vi "cs-scanning_v2.vi"() -> ()   [LabVIEW 2017]
uses:
  controls/boolean_info.ctl
  z-axis-params.ctl
  <vilib>/rvi/Emulation/niFpgaGetClockAttributes.vi
  <vilib>/rvi/Emulation/niFpgaSctlEmulationGetInTimedLoop.vi
  <vilib>/rvi/Emulation/niFpgaEmulationReportErrorSimple.vi
  <vilib>/rvi/Emulation/niFpgaProcessEmulError.vi
  <vilib>/rvi/eio/common/nirviEmuTemplateMethod_errors.vi
  <vilib>/rvi/Emulation/niFpgaEmulationIsFPGAContextNoSignature.vi
  <vilib>/rvi/DataTransferAndStorage/Container/Common/niFpgaContainerGetUniqueNameForEmu.vi
  <vilib>/rvi/Memory/Memory_Emulation/niFpgaMemoryEmulationCacheClearOnFirstRun.vi
  <vilib>/rvi/Memory/Memory_Emulation/nirvimemoryEmulationManagerCache_MakeExclusive.vi
  <vilib>/rvi/Memory/Memory_Emulation/niFpgaMemoryEmulationValidateCache.vi
  <vilib>/rvi/Memory/Memory_Emulation/nirvimemoryEmulationManagerCache_InsertValue.vi
  <vilib>/Utility/error.llb/Clear Errors.vi
  <vilib>/rvi/Memory/Memory_Emulation/nirvimemoryEmulationManagerCache_ReleaseExclusive.vi
  <vilib>/rvi/Memory/Memory_Emulation/nirvimemoryEmulationManagerCache_GetValue.vi
  <vilib>/rvi/Memory/Memory_Emulation/nirvimemoryEmulationManagerCache_SetValue.vi
  <vilib>/rvi/Emulation/niFpgaCriticalErrorInLSC.vi
  <vilib>/eio/EIONode/EIONode.xnode
  <vilib>/rvi/DataTransferAndStorage/Container/XNode/niFpgaContainer.xnode
  <vilib>/rvi/DataTransferAndStorage/Register/Emulation/niFpgaRegisterEmulation.vi
  FPGA-data-logging.lvlib
  libimaging-cs.lvlib
panel:
  out "stop_loops":bool
  out "xy_k":fxp<+/-,16,5>[](array[numeric])
  out "xy_ref":fxp<+/-,16,5>[](array[numeric])
  out "u_x saturated":bool
  out "u_y saturated":bool
  in  "Kiz_down":sgl format="%#_13g"
  in  "max_Z_settle_samples":i16
  in  "step_down_frac":fxp<+,8,1>
  out "state1-count":u64
  out "state5-count":u64
  out "state4-count":u64
  out "state3-count":u64
  out "state2-count":u64
  in  "collect all":bool
  in  "collect move":bool=TRUE
  out "iter":i32
  out "entity-index":i16
  in  "TsTicks":u32=1600
  in  "z-axis-params":T1={"TOL"=0.3, "ramp_rate"=0.0, "z_u_max"=5.0, "setpoint"=0.0, "Ki"=0.001, "Z_error_threshold"=0.0, "Z_settled_samples_threshold "=0, "z_UP"=0.0, "zup_N"=0, "TF Order"=2, "Num"=[-0.00254, 0.000408, 0.00295, 0.0, 0.0, 0.0, 0.0, 0.0, 0.0], "Den"=[0.982758, -1.98194, 1.0, 0.0, 0.0, 0.0, 0.0, 0.0, 0.0]} {"Z_error_threshold" format="%#_13g"; "ramp_rate" format="%#_13g"; "TOL" format="%#_13g"}
  out "number-settled-samples-Z":i16
  out "Current Case":u8
  out "boolean \nindicators":T2
  out "z-u(k)":sgl
  in  "ABORT":bool
  out "read fifo timeout":bool
  in  "numEntities":i16
  in  "init Z up":fxp<+/-,16,5>
  in  "trigger-0":bool
  out "number-settled-samples-y":i16
  out "number-settled-samples-x":i16
  in  "xy-error-threshold":sgl format="%#_13g"
  in  "settled-samples\nthreshold":i16
  in  "Ki-xy":sgl=0.001 format="%#_13g"
  in  "xy-bound":sgl
  in  "initial case":u8
  # "- If collect all = fasle and collect move = false,\nwe only collect measurement data.\n- If collect all = false, and collect move = true,\nwe collect measurement and move data.\n- If collect all = true, we collect everything."
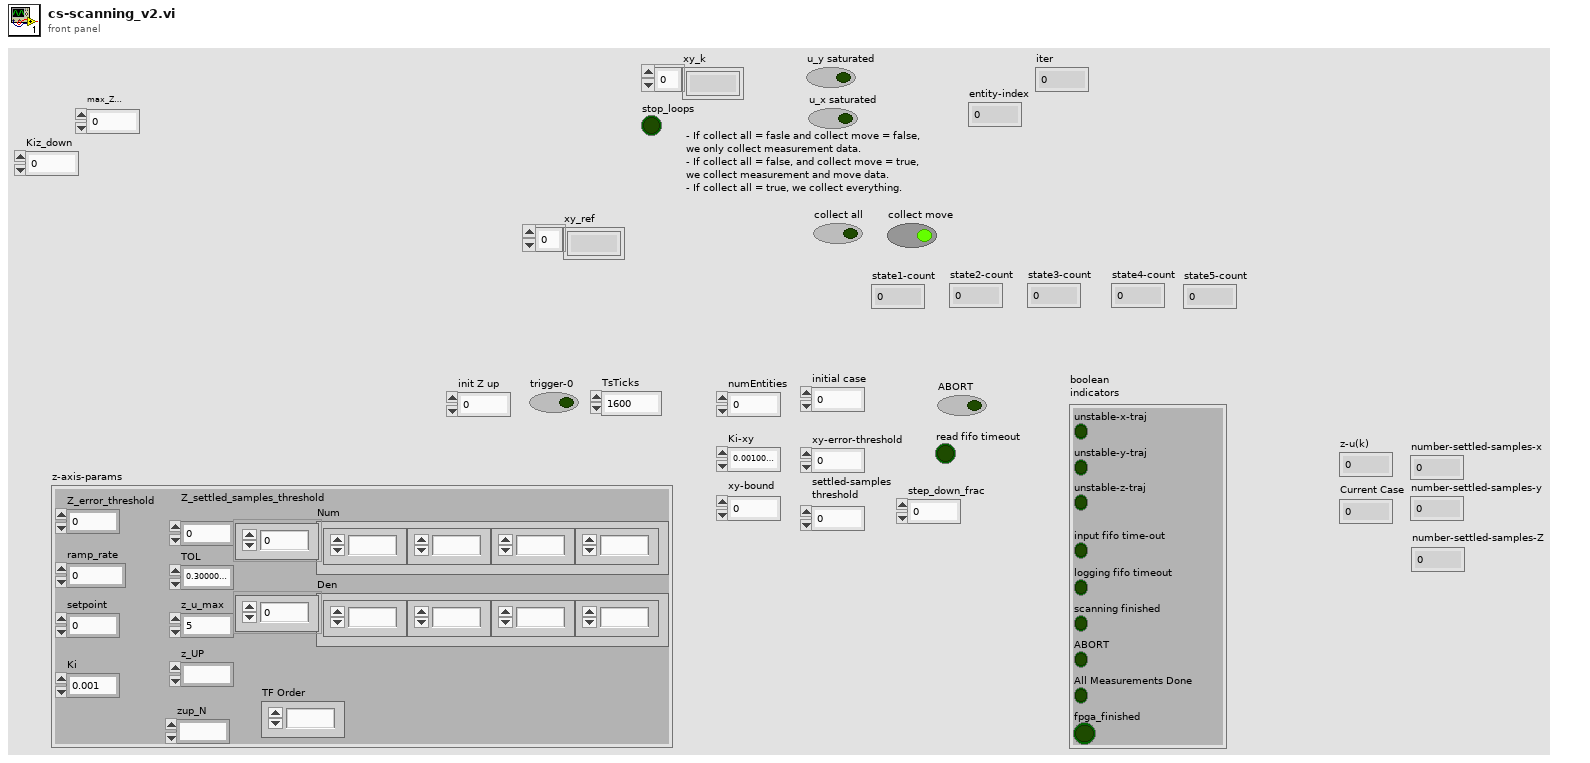
[diagram p1: front panel]
types:
  T1 = typedef "z-axis-params.ctl" = cluster{"TOL":sgl, "ramp_rate":sgl, "z_u_max":sgl, "setpoint":sgl, "Ki":sgl, "Z_error_threshold":sgl, "Z_settled_samples_threshold ":i16, "z_UP":fxp<+/-,16,5>, "zup_N":i16, "TF Order":i32, "Num":sgl[], "Den":sgl[]}
  T2 = typedef "boolean_info.ctl" = cluster{"unstable-z-traj":bool, "input fifo time-out":bool, "logging fifo timeout":bool, "scanning finished":bool, "unstable-x-traj":bool, "unstable-y-traj":bool, "ABORT":bool, "All Measurements Done":bool, "fpga_finished":bool}
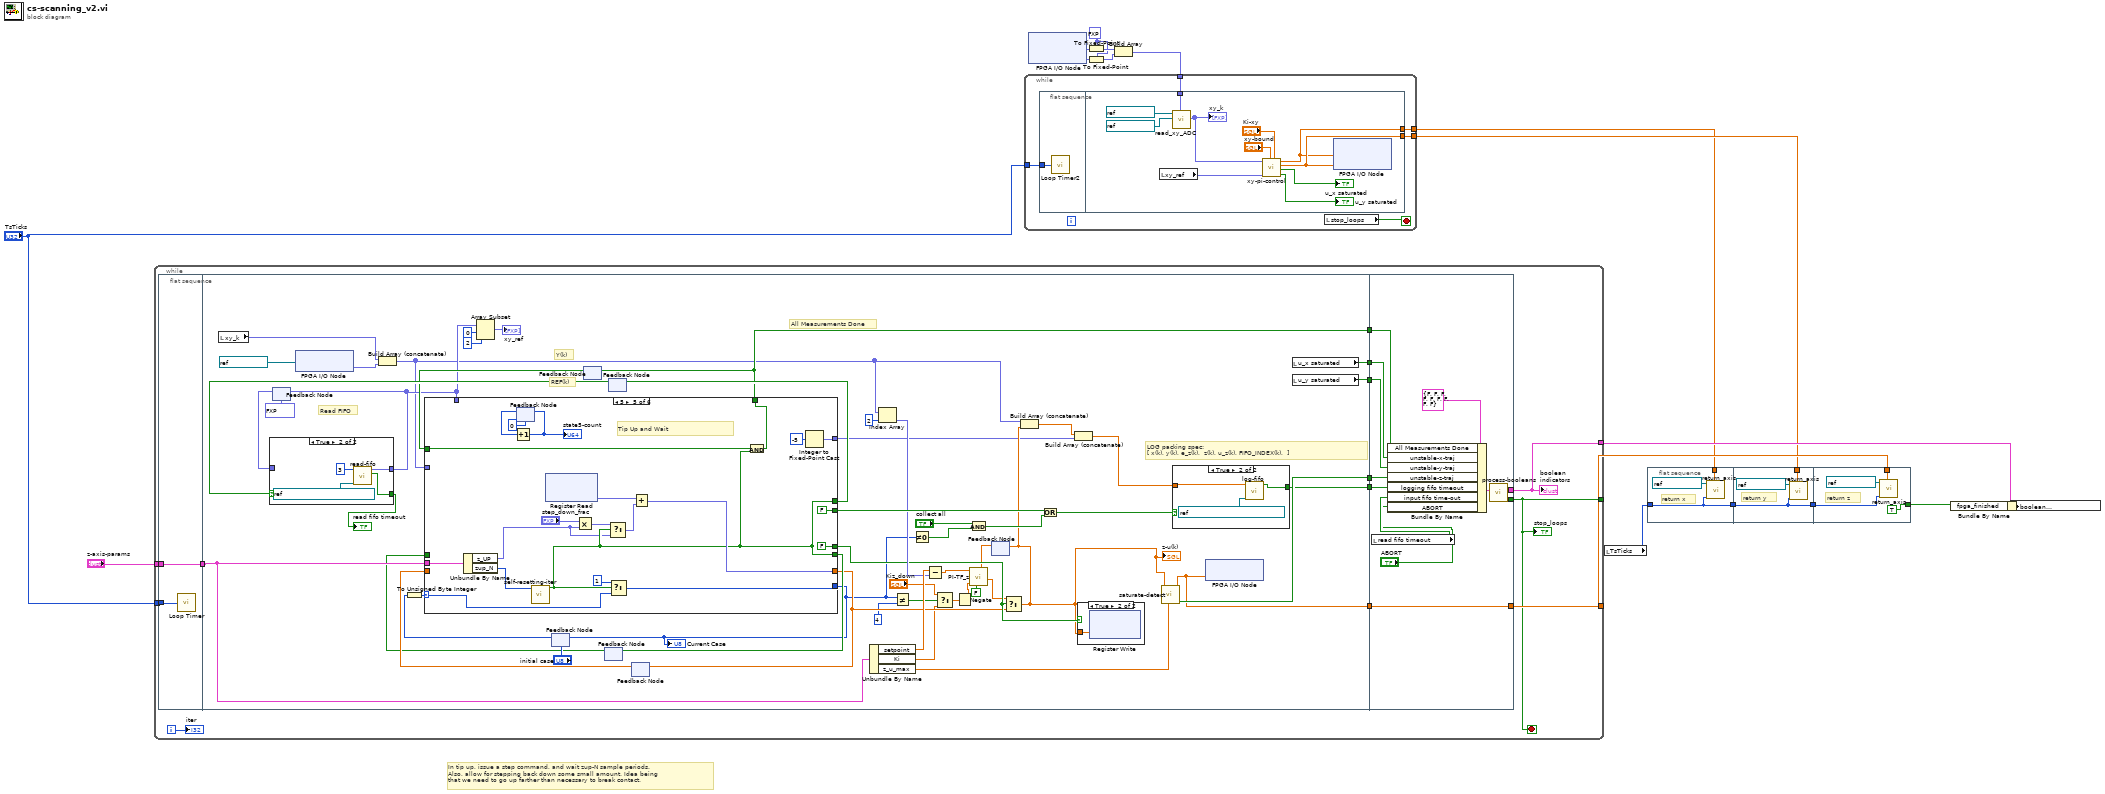
[diagram p0: block diagram]
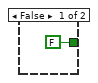
[diagram p3: hidden frame]
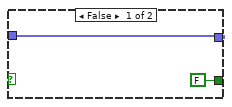
[diagram p4: hidden frame]
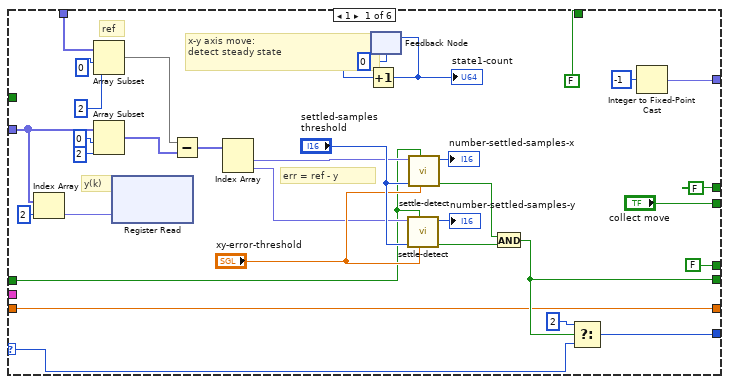
[diagram p5: hidden frame]
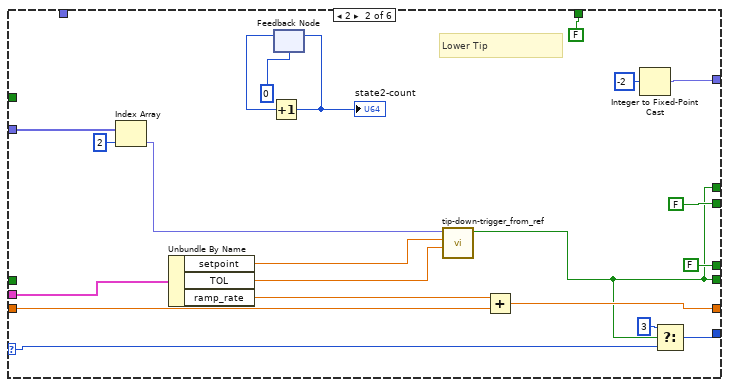
[diagram p6: hidden frame]
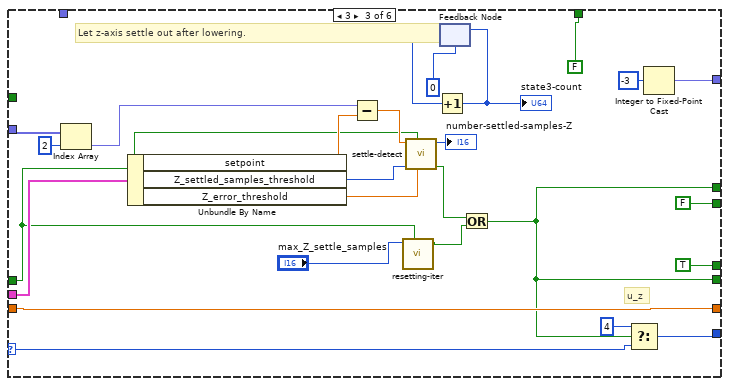
[diagram p7: hidden frame]
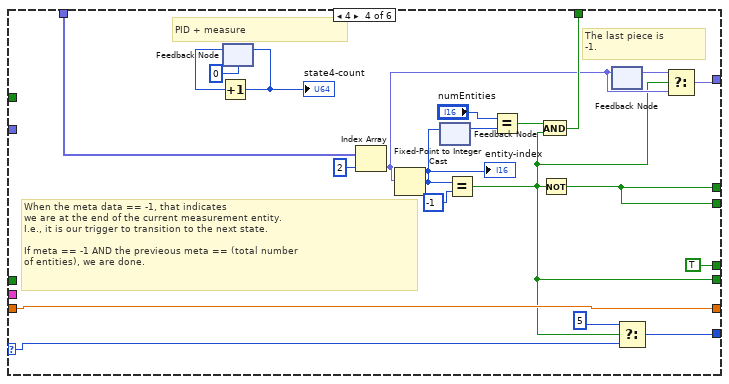
[diagram p8: hidden frame]
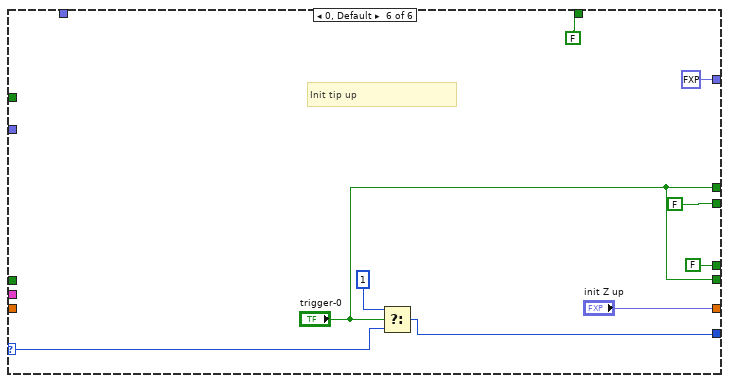
[diagram p9: hidden frame]
diagram:
  w13 = fxp<+/-,16,5> 0.0 ("fixed-point type")
  # "In tip up, issue a step command, and wait zup-N sample periods.\nAlso, allow for stepping back down some small amount. Idea being \nthat we need to go up farther than necessary to break contact."
  n1 = while {
    tunnel: "z-axis-params" -> [w26]
    tunnel: "TsTicks" -> [w25]
    tunnel: [w20] -> _
    tunnel: [w23] -> w8
    tunnel: [w21] -> w7
    i -> [w22]
    stop <- w20 stop-if-true
    n2 = flat-sequence {
      tunnel: w25 -> [w31]
      tunnel: w26 -> [w32]
      tunnel: [w32] -> w30
      tunnel: w30 -> [w74]
      tunnel: [w81] -> w29
      tunnel: [w80] -> w28
      tunnel: [w65] -> w27
      tunnel: [w75] -> w24
      tunnel: [w45] -> w19
      tunnel: [w44] -> w18
      tunnel: w29 -> [w240]
      tunnel: w28 -> [w237]
      tunnel: w27 -> [w234]
      tunnel: [w233] -> w20
      tunnel: [w232] -> w21
      tunnel: [w231] -> w23
      tunnel: w24 -> [w231]
      tunnel: w19 -> [w230]
      tunnel: w18 -> [w229]
      frame #0 {
        n3 = call "Loop Timer"("Count(Ticks)"=w31) -> ()  [unwired: 1 out]
      }
      frame #1 {
        # "All Measurements Done"
        # "REF(k)"
        # "Y(k)"
        # "LOG packing spec:\n[ x(k), y(k), e_z(k),  z(k), u_z(k), FIFO_INDEX(k),  ]"
        # "Read FIFO"
        n4 = local read "xy_k"() -> (w35:fxp<+/-,16,5>[])
        n5 = feedback #1(fxp<+/-,16,5>[] [0.0, 0.0, 0.0] ("unpacked-data")) -> (w84:fxp<+/-,16,5>[])
        n6 = xnode "FPGA I/O Node"("FPGA I/O In"=refnum<k21> "Mod2/AI2" ("y - ADC")) -> ("I/O Item"=w40:fxp<+/-,24,5>)  [unwired: 1 out]
        n7 = Build Array (concatenate)(w35, w40) -> (w39:fxp<+/-,24,5>[])
        n8 = feedback #2("initial case") -> (w33:u8)
        n9 = To Unsigned Byte Integer(number=w33) -> (unsigned 8bit integer=w34:u8)
        n10 = feedback #3() -> (w73:bool)  [unwired: 1 in]
        n11 = feedback #4() -> (w71:bool)  [unwired: 1 in]
        n12 = feedback #5() -> (w77:bool)  [unwired: 1 in]
        n13 = case shown="True" w77 {
          tunnel: w84 -> [w92 _]
          tunnel: [w92 w94] -> w41
          tunnel: [FALSE ("timout?") w93] -> w79
          frame False {
          }
          frame True {
            n14 = call "read-fifo.vi"("FIFO In"=refnum<k21> "host-to-fpga-fxp-16-5", "numChan"=3) -> ("timout?"=w93:bool, "unpacked-data"=w94:fxp<+/-,16,5>[])  [unwired: 8 in]
          }
        }
        "read fifo timeout" <- w79
        n15 = feedback-in #1(w41) -> ()
        n16 = Array Subset(array=w41, index=0, length=2) -> (→"xy_ref":fxp<+/-,16,5>[])
        n17 = feedback #6() -> (w83:sgl)  [unwired: 1 in]
        n18 = case shown="5" w34 {
          selector: w34 -> [w122 w150 w170 w196 w218 w226]
          tunnel: ["collect move" FALSE FALSE ("trigger-0") w188 FALSE FALSE] -> w66
          tunnel: [w123 w145 w171 w197 w217 w228] -> w54
          tunnel: w39 -> [w97 w147 w175 _ _ _]
          tunnel: [FALSE w132 w155 w188 w203 "trigger-0"] -> w78
          tunnel: [w102 w136 w157 w182 w207 "init Z up"] -> w55
          tunnel: w83 -> [w102 w143 w157 w182 _ _]
          tunnel: w74 -> [_ w149 w168 _ w214 _]
          tunnel: [FALSE FALSE FALSE w187 w199 FALSE] -> w65
          tunnel: w41 -> [w113 _ _ w190 _ _]
          tunnel: w73 -> [_ _ _ _ w212 _]
          tunnel: w71 -> [w111 _ w152 _ _ _]
          tunnel: [w109 w132 w155 w178 w203 "trigger-0"] -> w72
          tunnel: [FALSE ("trigger-0") FALSE ("trigger-0") TRUE ("trigger-0") TRUE ("trigger-0") FALSE ("trigger-0") FALSE ("trigger-0")] -> w61
          tunnel: [w100 w133 w159 w181 w201 fxp<+/-,16,5> 0.0 ("Element")] -> w36
          frame 1 {
            # "y(k)"
            # "err = ref - y"
            # "ref"
            # "x-y axis move: \ndetect steady state"
            n19 = Index Array(array=w97, index=2) -> (element=w99:fxp<+/-,24,5>)
            n20 = Array Subset(array=w113, index=0, length=2) -> (w117:fxp<+/-,16,5>[])
            n21 = Array Subset(array=w97, index=0, length=2) -> (w116:fxp<+/-,24,5>[])
            n22 = xnode ("Register Read")("Data"=w99) -> ()  [unwired: 1 in, 1 out]
            n23 = Subtract(x=w117, y=w116) -> (x-y=w108:fxp<+/-,25,6>[])
            n24 = Index Array(array=w108) -> (element #1=w115:fxp<+/-,25,6>, element #2=w114:fxp<+/-,25,6>)  [unwired: 2 in]
            n25 = feedback #7(u64 0) -> (w105:u64)
            n26 = Increment(x=w105) -> (x+1=w106:u64)
            "state1-count" <- w106
            n27 = feedback-in #7(w106) -> ()
            n28 = call "settle-detect.vi"("error-max"="xy-error-threshold", "reset"=w111, "settled-samples\nthreshold"="settled-samples\nthreshold", "err(k)"=w114) -> ("has-settled"=w130:bool, "number-settled-samples"=→"number-settled-samples-y":u16)  [unwired: 6 in]
            n29 = call "settle-detect.vi"("error-max"="xy-error-threshold", "reset"=w111, "settled-samples\nthreshold"="settled-samples\nthreshold", "err(k)"=w115) -> ("has-settled"=w129:bool, "number-settled-samples"=→"number-settled-samples-x":u16)  [unwired: 6 in]
            n30 = And(x=w129, y=w130) -> (x .and. y?=w109:bool)
            n31 = Select(t=u8 2, s=w109, f=w122) -> (s? t:f=w123:u8)
            n32 = Integer to Fixed-Point Cast(integer=i16 -1) -> (fixed-point=w100:fxp<+/-,16,5>)  [unwired: 1 in]
          }
          frame 2 {
            # "Lower Tip"
            n33 = Index Array(array=w147, index=2) -> (element=w146:fxp<+/-,24,5>)
            n34 = Unbundle By Name(w149) -> ("setpoint"=w135:sgl, "TOL"=w131:sgl, "ramp_rate"=w151:sgl)
            n35 = feedback #8(u64 0) -> (w139:u64)
            n36 = Increment(x=w139) -> (x+1=w140:u64)
            "state2-count" <- w140
            n37 = feedback-in #8(w140) -> ()
            n38 = call "tip-down-trigger_from_ref.vi"("TOL"=w131, "setpoint"=w135, "I/O Item"=w146) -> ("Boolean"=w132:bool)  [unwired: 8 in]
            n39 = Add(x=w151, y=w143) -> (x+y=w136:sgl)
            n40 = Integer to Fixed-Point Cast(integer=i16 -2) -> (fixed-point=w133:fxp<+/-,16,5>)  [unwired: 1 in]
            n41 = Select(t=u8 3, s=w132, f=w150) -> (s? t:f=w145:u8)
          }
          frame 3 {
            # "u_z"
            # "Let z-axis settle out after lowering."
            n42 = Index Array(array=w175, index=2) -> (element=w173:fxp<+/-,24,5>)
            n43 = Unbundle By Name(w168) -> ("setpoint"=w158:sgl, "Z_settled_samples_threshold"=w167:i16, "Z_error_threshold"=w166:sgl)
            n44 = Subtract(x=w173, y=w158) -> (x-y=w176:sgl)
            n45 = call "resetting-iter.vi"("reset"=w152, "N"="max_Z_settle_samples") -> ("Boolean"=w154:bool)  [unwired: 8 in, 1 out]
            n46 = call "settle-detect.vi"("error-max"=w166, "reset"=w152, "settled-samples\nthreshold"=w167, "err(k)"=w176) -> ("has-settled"=w156:bool, "number-settled-samples"=→"number-settled-samples-Z":u16)  [unwired: 6 in]
            n47 = feedback #9(u64 0) -> (w163:u64)
            n48 = Increment(x=w163) -> (x+1=w164:u64)
            "state3-count" <- w164
            n49 = feedback-in #9(w164) -> ()
            n50 = Or(x=w156, y=w154) -> (x .or. y?=w155:bool)
            n51 = Select(t=u8 4, s=w155, f=w170) -> (s? t:f=w171:u8)
            n52 = Integer to Fixed-Point Cast(integer=i16 -3) -> (fixed-point=w159:fxp<+/-,16,5>)  [unwired: 1 in]
          }
          frame 4 {
            # "The last piece is\n-1."
            # "When the meta data == -1, that indicates\nwe are at the end of the current measurement entity.\nI.e., it is our trigger to transition to the next state.\n\nIf meta == -1 AND the previeous meta == (total number\nof entities), we are done."
            # "PID + measure"
            n53 = feedback #10(u64 0) -> (w185:u64)
            n54 = Increment(x=w185) -> (x+1=w186:u64)
            "state4-count" <- w186
            n55 = feedback-in #10(w186) -> ()
            n56 = Index Array(array=w190, index=2) -> (element=w179:fxp<+/-,16,5>)
            n57 = Fixed-Point to Integer Cast(1:w179) -> (0:w189:i16)
            "entity-index" <- w189
            n58 = feedback #11() -> (w191:i16)  [unwired: 1 in]
            n59 = feedback-in #11(w189) -> ()
            n60 = Equal?(x=w189, y=i16 -1) -> (x = y?=w178:bool)
            n61 = Equal?(x="numEntities", y=w191) -> (x = y?=w192:bool)
            n62 = And(x=w192, y=w178) -> (x .and. y?=w187:bool)
            n63 = Not(x=w178) -> (.not. x?=w188:bool)
            n64 = feedback #12() -> (w180:fxp<+/-,16,5>)  [unwired: 1 in]
            n65 = feedback-in #12(w179) -> ()
            n66 = Select(t=u8 5, s=w178, f=w196) -> (s? t:f=w197:u8)
            n67 = Select(t=w180, s=w178, f=w179) -> (s? t:f=w181:fxp<+/-,16,5>)
          }
          frame 5 {
            # "Tip Up and Wait"
            n68 = Unbundle By Name(w214) -> ("z_UP"=w202:fxp<+/-,16,5>, "zup_N"=w213:i16)
            n69 = feedback #13(u64 0) -> (w210:u64)
            n70 = Increment(x=w210) -> (x+1=w211:u64)
            "state5-count" <- w211
            n71 = feedback-in #13(w211) -> ()
            n72 = call "self-resetting-iter.vi"("N"=w213) -> ("Boolean"=w203:bool)  [unwired: 9 in, 1 out]
            n73 = xnode ("Register Read")() -> ("Data"=w215:fxp<+/-,16,5>)  [unwired: 1 in, 1 out]
            n74 = Multiply(x="step_down_frac", y=w202) -> (x*y=w206:fxp<+/-,24,6>)
            n75 = Select(t=w206, s=w203, f=w202) -> (s? t:f=w204:fxp<+/-,24,6>)
            n76 = Select(t=u8 1, s=w203, f=w218) -> (s? t:f=w217:u8)
            n77 = Add(x=w215, y=w204) -> (x+y=w207:fxp<+/-,25,7>)
            n78 = And(x=w212, y=w203) -> (x .and. y?=w199:bool)
            n79 = Integer to Fixed-Point Cast(integer=i16 -5) -> (fixed-point=w201:fxp<+/-,16,5>)  [unwired: 1 in]
          }
          frame 0, Default {
            # "Init tip up"
            n80 = Select(t=u8 1, s="trigger-0", f=w226) -> (s? t:f=w228:u8)
          }
        }
        "Current Case" <- w54
        n81 = feedback-in #2(w54) -> ()
        n82 = feedback-in #3(w65) -> ()
        n83 = feedback-in #4(w72) -> ()
        n84 = feedback-in #5(w78) -> ()
        n85 = feedback-in #6(w55) -> ()
        n86 = Unbundle By Name(w74) -> ("setpoint"=w64:sgl, "Ki"=w48:sgl, "z_u_max"=w60:sgl)
        n87 = Index Array(array=w39, index=2) -> (element=w62:fxp<+/-,24,5>)
        n88 = Not Equal?(x=w54, y=u8 4) -> (x != y?=w51:bool)
        n89 = Not Equal To 0?(x=w54) -> (x != 0?=w69:bool)
        n90 = Subtract(x=w64, y=w62) -> (x-y=w59:sgl)
        n91 = Select(t="Kiz_down", s=w51, f=w48) -> (s? t:f=w50:sgl)
        n92 = Negate(x=w50) -> (-x=w49:sgl)
        n93 = And(x="collect all", y=w69) -> (x .and. y?=w67:bool)
        n94 = feedback #14() -> (w56:sgl)  [unwired: 1 in]
        n95 = call "PI-TF_z.vi"("u(k-1)"=w56, "reset"=FALSE, "Ki"=w49, "e(k)"=w59) -> ("u(k)"=w57:sgl)  [unwired: 7 in]
        n96 = Select(t=w57, s=w61, f=w55) -> (s? t:f=w37:sgl)
        "z-u(k)" <- w37
        n97 = feedback-in #14(w37) -> ()
        n98 = Build Array (concatenate)(w39, w37) -> (w38:sgl[])
        n99 = Or(x=w66, y=w67) -> (x .or. y?=w70:bool)
        n100 = Build Array (concatenate)(w38, w36) -> (w82:sgl[])
        n101 = case shown="True" w61 {
          tunnel: w37 -> [_ w86]
          frame False {
          }
          frame True {
            n102 = xnode ("Register Write")("Data"=w86) -> ()  [unwired: 1 in, 1 out]
          }
        }
        n103 = call "saturate-detect.vi"("bound"=w60, "x"=w37) -> ("saturated"=w81:bool, "sat(x)"=w75:sgl)  [unwired: 8 in]
        n104 = case shown="True" w70 {
          tunnel: w82 -> [_ w89]
          tunnel: [FALSE ("logging-timeout?") w88] -> w80
          frame False {
          }
          frame True {
            n105 = call "log-fifo.vi"("FIFO In"=refnum<k21> "fpga-to-host2-fxp-16-5", "input-data"=w89) -> ("logging-timeout?"=w88:bool)  [unwired: 9 in]
          }
        }
        n106 = xnode "FPGA I/O Node"("Mod1/AO2"=w75) -> ()  [unwired: 1 in, 1 out]
        n107 = local read "u_x saturated"() -> (w45:bool)
        n108 = local read "u_y saturated"() -> (w44:bool)
      }
      frame #2 {
        n109 = local read "read fifo timeout"() -> (w236:bool)
        n110 = Bundle By Name(cluster=T2 {"unstable-z-traj"=FALSE, "input fifo time-out"=FALSE, "logging fifo timeout"=FALSE, "scanning finished"=FALSE, "unstable-x-traj"=FALSE, "unstable-y-traj"=FALSE, "ABORT"=FALSE, "All Measurements Done"=FALSE, "fpga_finished"=FALSE} ("boolean errors"), "All Measurements Done"=w234, "unstable-x-traj"=w230, "unstable-y-traj"=w229, "unstable-z-traj"=w240, "logging fifo timeout"=w237, "input fifo time-out"=w236, "ABORT"="ABORT") -> (w238:T2)
        n111 = call "process-booleans.vi"("boolean indicators 2"=w238) -> ("scaning finished"=w233:bool, "boolean indicators"=w232:T2)  [unwired: 9 in]
      }
    }
    "boolean \nindicators" <- w21
    "iter" <- w22
    "stop_loops" <- w20
  }
  n112 = xnode "FPGA I/O Node"() -> ("Mod2/AI0"=w16:fxp<+/-,24,5>, "Mod2/AI1"=w14:fxp<+/-,24,5>)  [unwired: 2 in, 2 out]
  n113 = To Fixed-Point(fixed-point type=w13, number=w16) -> (fixed-point=w17:fxp<+/-,16,5>)
  n114 = To Fixed-Point(fixed-point type=w13, number=w14) -> (fixed-point=w15:fxp<+/-,16,5>)
  n115 = Build Array(w17, w15) -> (w1:fxp<+/-,16,5>[])
  n116 = while {
    tunnel: "TsTicks" -> [w245]
    tunnel: [w244] -> w3
    tunnel: [w243] -> w2
    tunnel: w1 -> [w242]
    stop <- w241 stop-if-true
    n117 = flat-sequence {
      tunnel: w245 -> [w246]
      tunnel: [w256] -> w244
      tunnel: [w255] -> w243
      tunnel: w242 -> [w251]
      frame #0 {
        n118 = call "Loop Timer2"("Count(Ticks)"=w246) -> ()  [unwired: 1 out]
      }
      frame #1 {
        n119 = local read "xy_ref"() -> (w248:fxp<+/-,16,5>[])
        n120 = call "read_xy_ADC.vi"("x(0), y(0)"=w251, "y - ADC"=refnum<k21> "Mod2/AI1", "x - ADC"=refnum<k21> "Mod2/AI0") -> ("x_y"=w247:fxp<+/-,17,6>[])  [unwired: 8 in]
        "xy_k" <- w247
        n121 = call "xy-pi-control.vi"("Ki-xy"="Ki-xy", "xy-umax"="xy-bound", "xy-ref"=w248, "x_k-y_k"=w247) -> ("u_y saturated"=→"u_y saturated":bool, "u_x saturated"=→"u_x saturated":bool, "sat(u_y)"=w256:sgl, "sat(u_x)"=w255:sgl)  [unwired: 4 in]
        n122 = xnode "FPGA I/O Node"("Mod1/AO0"=w255, "Mod1/AO1"=w256) -> ()  [unwired: 2 in, 2 out]
      }
    }
    n123 = local read "stop_loops"() -> (w241:bool)
  }
  n124 = local read "TsTicks"() -> (w9:u32)
  n125 = flat-sequence {
    tunnel: w9 -> [w259]
    tunnel: w2 -> [w260]
    tunnel: [w259] -> w11
    tunnel: w3 -> [w263]
    tunnel: w11 -> [w261]
    tunnel: [w261] -> w10
    tunnel: w8 -> [w267]
    tunnel: w10 -> [w265]
    tunnel: [TRUE] -> w6
    frame #0 {
      # "return x"
      n126 = call "return_axis.vi"("u(0)"=w260, "TsTicks"=w259, "FPGA I/O In"=refnum<k21> "Mod1/AO0") -> ()  [unwired: 9 in]
    }
    frame #1 {
      # "return y"
      n127 = call "return_axis.vi"("u(0)"=w263, "TsTicks"=w261, "FPGA I/O In"=refnum<k21> "Mod1/AO1") -> ()  [unwired: 9 in]
    }
    frame #2 {
      # "return z"
      n128 = call "return_axis.vi"("u(0)"=w267, "TsTicks"=w265, "FPGA I/O In"=refnum<k21> "Mod1/AO2") -> ()  [unwired: 9 in]
    }
  }
  n129 = Bundle By Name(cluster=w7, "fpga_finished"=w6) -> (w5:T2)
  n130 = local write "boolean \nindicators"(w5) -> ()
